vi "DestroyParser.vi"(8 "error in (no error)":errorcluster, 11 "ArgumentParser in":refnum<class "ArgumentParser.lvclass">) -> (0 "error out":errorcluster, 3 "ArgumentParser out":refnum<class "ArgumentParser.lvclass">)   [LabVIEW 2022 SP3, in "ArgumentParser.lvlib" / "ArgumentParser.lvclass"]
uses:
  ArgumentParser.lvclass
  ArgumentParser.lvclass/ArgumentParser.ctl
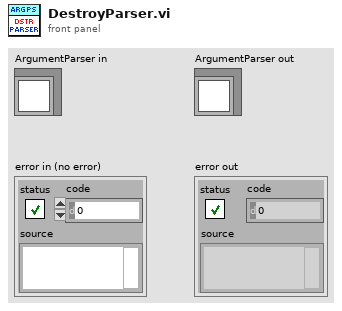
[diagram p1: front panel]
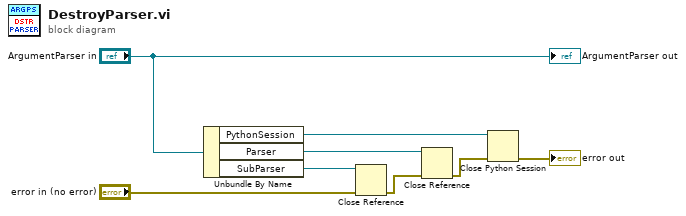
[diagram p0: block diagram]
diagram:
  n1 = Unbundle By Name("ArgumentParser in") -> ("PythonSession"=w5:refnum<k35>, "Parser"=w6:refnum<k38>, "SubParser"=w7:refnum<k38>)
  n2 = Close Reference(reference=w7, error in (no error)="error in (no error)") -> (error out=w2:errorcluster)
  n3 = Close Reference(reference=w6, error in (no error)=w2) -> (error out=w1:errorcluster)
  n4 = Close Python Session(session in=w5, error in=w1) -> (11:→"error out":errorcluster)
  "ArgumentParser out" <- "ArgumentParser in"
